vi "Read Array.vi"(11 "Ordered Array.lvclass in":refnum<class "Ordered Array.lvclass">) -> (2 "Array":u32[](array[numeric]), 3 "Ordered Array.lvclass out":refnum<class "Ordered Array.lvclass">)   [LabVIEW 2011, in "Ordered Array.lvclass"]
uses:
  Ordered Array.lvclass
  Ordered Array.lvclass/Ordered Array.ctl
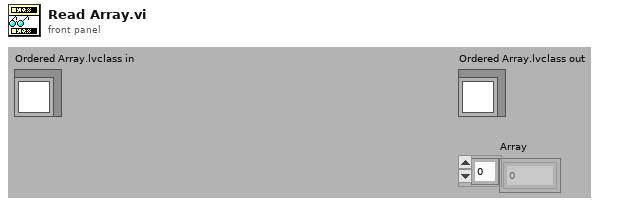
[diagram p1: front panel]
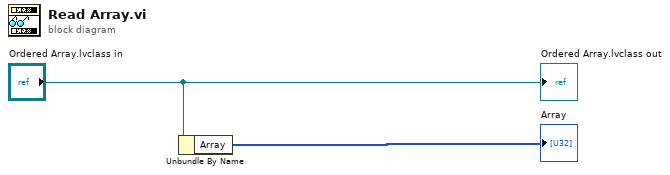
[diagram p0: block diagram]
diagram:
  n1 = Unbundle By Name("Ordered Array.lvclass in") -> ("Array"=→"Array":u32[])
  "Ordered Array.lvclass out" <- "Ordered Array.lvclass in"
